vi "NeoPixelShow.vi"(8 "error in (no error)":errorcluster, 11 "AdaFruit-Seesaw in":refnum<class "AdaFruit-Seesaw.lvclass">) -> (0 "error out":errorcluster, 3 "AdaFruit-Seesaw out":refnum<class "AdaFruit-Seesaw.lvclass">)   [LabVIEW 2020, in "CTI-Peripheral.lvlib" / "AdaFruit-Seesaw.lvclass"]
uses:
  AdaFruit-Seesaw.lvclass
  Private/SeeSawBaseAddresses.ctl
  Private/SeeSawNEOPIXELFunctions.ctl
  AdaFruit-Seesaw.lvclass/AdaFruit-Seesaw.ctl
  CTI/I2C Connection/I2C Connection.lvclass/I2C Connection.ctl
  CTI/Session/I2C Write Data.vi
  CTI/I2C Connection/I2C Connection.lvclass
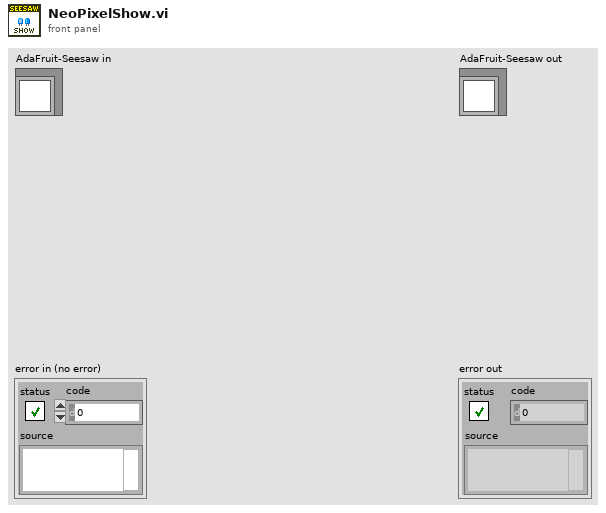
[diagram p1: front panel]
types:
  T1 = typedef "CTI-Peripheral.lvlib/AdaFruit-Seesaw.lvclass/SeeSawNEOPIXELFunctions.ctl" = u8
  T2 = typedef "CTI-Peripheral.lvlib/AdaFruit-Seesaw.lvclass/SeeSawBaseAddresses.ctl" = u8
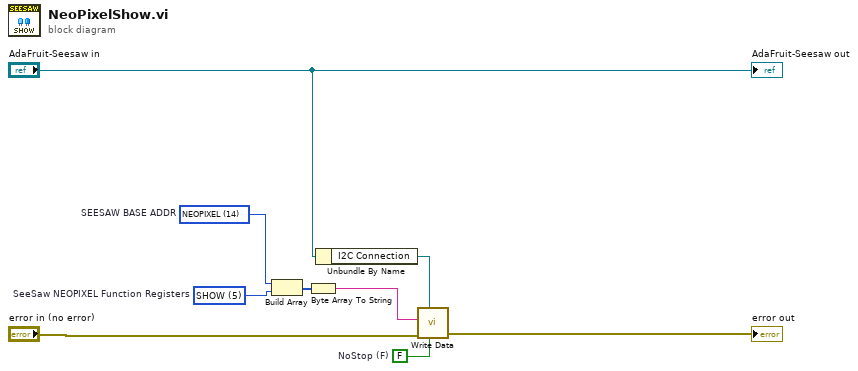
[diagram p0: block diagram]
diagram:
  w1 = T1 5 items=["STATUS", "PIN", "SPEED", "BUF_LENGTH", "BUF", "SHOW"]  # SeeSaw NEOPIXEL Function Registers
  w6 = FALSE  # NoStop (F)
  w9 = T2 14 items=["STATUS"=0, "GPIO"=1, "SERCOM0"=2, "TIMER"=8, "ADC"=9, "DAC"=10, "INTERUPT"=11, "DAP"=12, "EEPROM"=13, "NEOPIXEL"=14, "TOUCH"=15, "KEYPAD"=16, "ENCODER"=17, "SPECTRUM"=18]  # SEESAW BASE ADDR
  n1 = Build Array(w9, w1) -> (w8:T1[])
  n2 = Byte Array To String(unsigned byte array=w8) -> (string=w5:string)
  n3 = Unbundle By Name("AdaFruit-Seesaw in") -> ("I2C Connection"=w7:refnum<class "I2C Connection.lvclass">)
  n4 = call "Write Data.vi"("NoStop (F)"=w6, "I2C Connection"=w7, "error in (no error)"="error in (no error)", "Data"=w5) -> ("error out"=→"error out":errorcluster)  [unwired: 7 in]
  "AdaFruit-Seesaw out" <- "AdaFruit-Seesaw in"
